vi "Split_String.vi"(1 "TEXTO DE ENTRADA":string) -> (0 "VETOR":dbl[](array[numeric]))   [LabVIEW 2018]
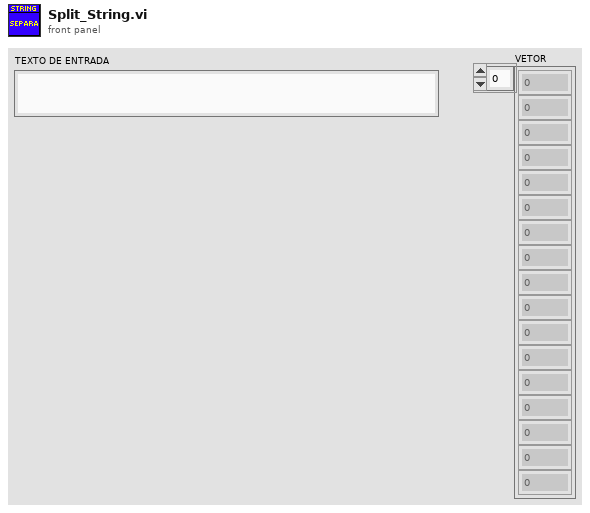
[diagram p1: front panel]
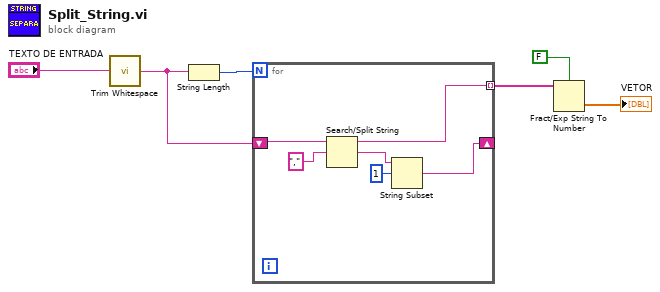
[diagram p0: block diagram]
diagram:
  n1 = call <vilib>:"Trim Whitespace.vi"("string"="TEXTO DE ENTRADA") -> ("trimmed string"=w4:string)  [unwired: 1 in]
  n2 = String Length(string=w4) -> (length=w5:i32)
  n3 = for {
    N: w5 -> [_]
    shift-right: [w8] -> _
    shift-left: w4 -> [w12]
    tunnel: [w7] -> w3 mode=indexing
    n4 = Search/Split String(string=w12, search string/char (-)=",") -> (substring before match=w7:string, match + rest of string=w10:string)  [unwired: 1 in, 1 out]
    n5 = String Subset(string=w10, offset (0)=1) -> (substring=w8:string)  [unwired: 1 in]
  }
  n6 = Fract/Exp String To Number(use system decimal point (T)=FALSE, string=w3) -> (number=→"VETOR":dbl[])  [unwired: 2 in, 1 out]
